vi "Fetch Measurement(Math).vi"(0 "VISA resource name":refnum<visa-resource-name>, 11 "error in (no error)":errorcluster) -> (3 "Maximum":dbl, 4 "VISA resource name out":refnum<visa-resource-name>, 6 "Count":dbl, 8 "Average":dbl, 10 "Standard Deviation":dbl, 14 "Minimum":dbl, 15 "error out":errorcluster)   [LabVIEW 2020, in "3458A Virtual Digitizer.lvlib" / "3458A Basic Driver.lvlib"]
doc: "Returns the statistics of measurements that are taken by the DMM after sample count has been set in the configure multipoint and the trigger count has been set in the Read Measurement Statistics VI.\n\n<B>Note:</B> Use this VI only with other low-level VIs. The high-level VIs automatically incorporate this functionality. This VI does not check the instrument status. If you want to check the instrument status, call the Error Query VI at the conclusion of the sequence."
uses:
  3458A Basic Driver.lvlib
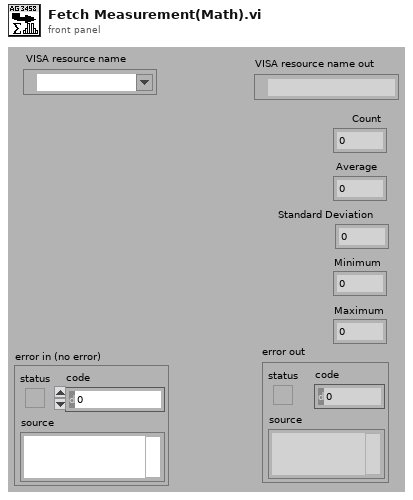
[diagram p1: front panel]
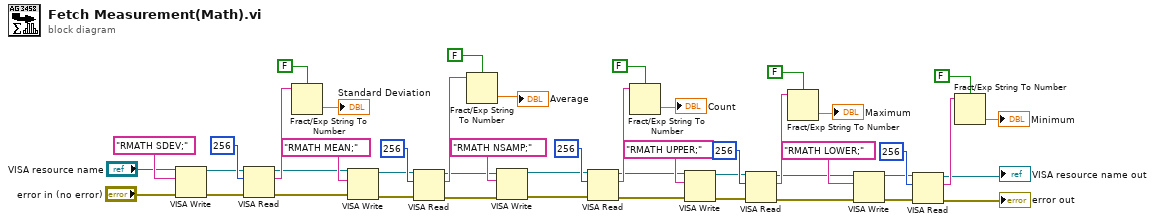
[diagram p0: block diagram]
diagram:
  n1 = VISA Write(VISA resource name="VISA resource name", write buffer="RMATH SDEV;", error in (no error)="error in (no error)") -> (VISA resource name out=w11:refnum<visa-resource-name>, error out=w10:errorcluster)  [unwired: 1 out]
  n2 = VISA Read(VISA resource name=w11, byte count=u32 256, error in (no error)=w10) -> (VISA resource name out=w28:refnum<visa-resource-name>, read buffer=w46:string, error out=w27:errorcluster)  [unwired: 1 out]
  n3 = Fract/Exp String To Number(use system decimal point (T)=FALSE, string=w46) -> (number=→"Standard Deviation":dbl)  [unwired: 2 in, 1 out]
  n4 = VISA Write(VISA resource name=w28, write buffer="RMATH MEAN;", error in (no error)=w27) -> (VISA resource name out=w43:refnum<visa-resource-name>, error out=w42:errorcluster)  [unwired: 1 out]
  n5 = VISA Read(VISA resource name=w43, byte count=u32 256, error in (no error)=w42) -> (VISA resource name out=w24:refnum<visa-resource-name>, read buffer=w25:string, error out=w23:errorcluster)  [unwired: 1 out]
  n6 = Fract/Exp String To Number(use system decimal point (T)=FALSE, string=w25) -> (number=→"Average":dbl)  [unwired: 2 in, 1 out]
  n7 = VISA Write(VISA resource name=w24, write buffer="RMATH NSAMP;", error in (no error)=w23) -> (VISA resource name out=w39:refnum<visa-resource-name>, error out=w38:errorcluster)  [unwired: 1 out]
  n8 = VISA Read(VISA resource name=w39, byte count=u32 256, error in (no error)=w38) -> (VISA resource name out=w20:refnum<visa-resource-name>, read buffer=w21:string, error out=w19:errorcluster)  [unwired: 1 out]
  n9 = Fract/Exp String To Number(use system decimal point (T)=FALSE, string=w21) -> (number=→"Count":dbl)  [unwired: 2 in, 1 out]
  n10 = VISA Write(VISA resource name=w20, write buffer="RMATH UPPER;", error in (no error)=w19) -> (VISA resource name out=w35:refnum<visa-resource-name>, error out=w34:errorcluster)  [unwired: 1 out]
  n11 = VISA Read(VISA resource name=w35, byte count=u32 256, error in (no error)=w34) -> (VISA resource name out=w16:refnum<visa-resource-name>, read buffer=w18:string, error out=w15:errorcluster)  [unwired: 1 out]
  n12 = Fract/Exp String To Number(use system decimal point (T)=FALSE, string=w18) -> (number=→"Maximum":dbl)  [unwired: 2 in, 1 out]
  n13 = VISA Write(VISA resource name=w16, write buffer="RMATH LOWER;", error in (no error)=w15) -> (VISA resource name out=w31:refnum<visa-resource-name>, error out=w30:errorcluster)  [unwired: 1 out]
  n14 = VISA Read(VISA resource name=w31, byte count=u32 256, error in (no error)=w30) -> (VISA resource name out=→"VISA resource name out":refnum<visa-resource-name>, read buffer=w13:string, error out=→"error out":errorcluster)  [unwired: 1 out]
  n15 = Fract/Exp String To Number(use system decimal point (T)=FALSE, string=w13) -> (number=→"Minimum":dbl)  [unwired: 2 in, 1 out]
